vi "Part 2.vi"(11 "Input":string) -> (3 "Output":i64)   [LabVIEW 2021]
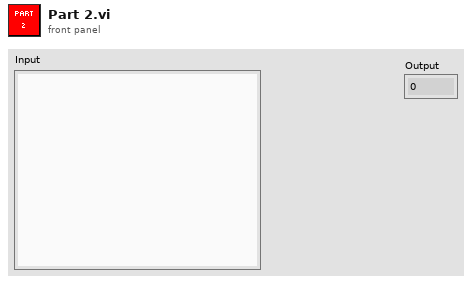
[diagram p1: front panel]
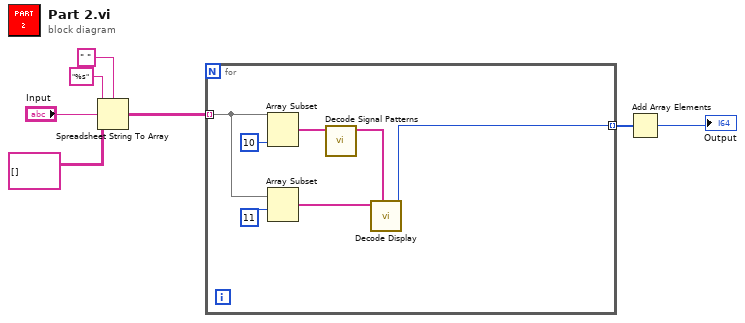
[diagram p0: block diagram]
diagram:
  n1 = Spreadsheet String To Array(delimiter (Tab)=" ", format string="%s", spreadsheet string="Input", array type (2D Dbl)=string[][] []) -> (array=w4:string[][])
  n2 = for {
    tunnel: w4 -> [w12] mode=indexing
    tunnel: [w8] -> w3 mode=indexing
    n3 = Array Subset(array=w12, length=10) -> (w13:string[])  [unwired: 1 in]
    n4 = Array Subset(array=w12, index=11 ("length")) -> (w10:string[])  [unwired: 1 in]
    n5 = call "Decode Signal Patterns.vi"("Signal Pattern"=w13) -> ("Segment Pattern"=w9:string[])  [unwired: 10 in]
    n6 = call "Decode Display.vi"("Segment Pattern"=w9, "Display"=w10) -> ("Value on Display"=w8:i64)  [unwired: 9 in]
  }
  n7 = Add Array Elements(numeric array=w3) -> (sum=→"Output":i64)
